vi "Autonomous Independent (Team 2175's conflicted copy 2013-08-08).vi"   [LabVIEW 2012]
doc: "This VI is called when autonomous begins, and will automatically be terminated when autonomous ends. You can carry out timed or sensor driven robot movement independently without needing to return to the caller."
uses:
  Robot Global Data.vi
  2013 Competition Code rev4 (Pre-Mariucci)/Auto Steer (Gyro).vi
types:
  T1 = typedef "WPI_GyroDevRef.ctl" = cluster{"DevStatus":errorcluster, "Analog Module":T2, "Analog Channel":T3, "Offset":dbl, "Gain (VoltsPerDegree/Second)":dbl}
  T2 = typedef "FPGA_TypedefAnalogModule.ctl" = enum16{"Analog Module 1", "Analog Module 2"}
  T3 = typedef "FPGA_AIChannel.ctl" = enum8{"AI 1", "AI 2", "AI 3", "AI 4", "AI 5", "AI 6", "AI 7", "AI 8", "Invalid"}
  T4 = typedef "WPI_EncoderDevRef.ctl" = cluster{"DevStatus":errorcluster, "EncoderIndex":T5, "CounterIndex":T6, "DistancePerCount":dbl, "Decoding Type":T7}
  T5 = typedef "FPGA_EncoderIdx.ctl" = enum8{"Enc 0", "Enc 1", "Enc 2", "Enc 3", "Invalid"}
  T6 = typedef "FPGA_CounterCtrSystemIndex.ctl" = enum8{"Ctr 0", "Ctr 1", "Ctr 2", "Ctr 3", "Ctr 4", "Ctr 5", "Ctr 6", "Ctr 7", "Invalid"}
  T7 = typedef "WPI_EncoderType.ctl" = enum16{"1x", "2x", "4x"}
  T8 = typedef "WPI_DigitalInputDevRef.ctl" = cluster{"DevStatus":errorcluster, "DIO Channel":T9, "Digital Module":T10}
  T9 = typedef "FPGA_DIOChannel.ctl" = enum8{"DIO 1", "DIO 2", "DIO 3", "DIO 4", "DIO 5", "DIO 6", "DIO 7", "DIO 8", "DIO 9", "DIO 10", "DIO 11", "DIO 12", "DIO 13", "DIO 14", "Invalid"}
  T10 = typedef "FPGA_TypedefDigitalModule.ctl" = enum16{"Digital Module 1", "Digital Module 2"}
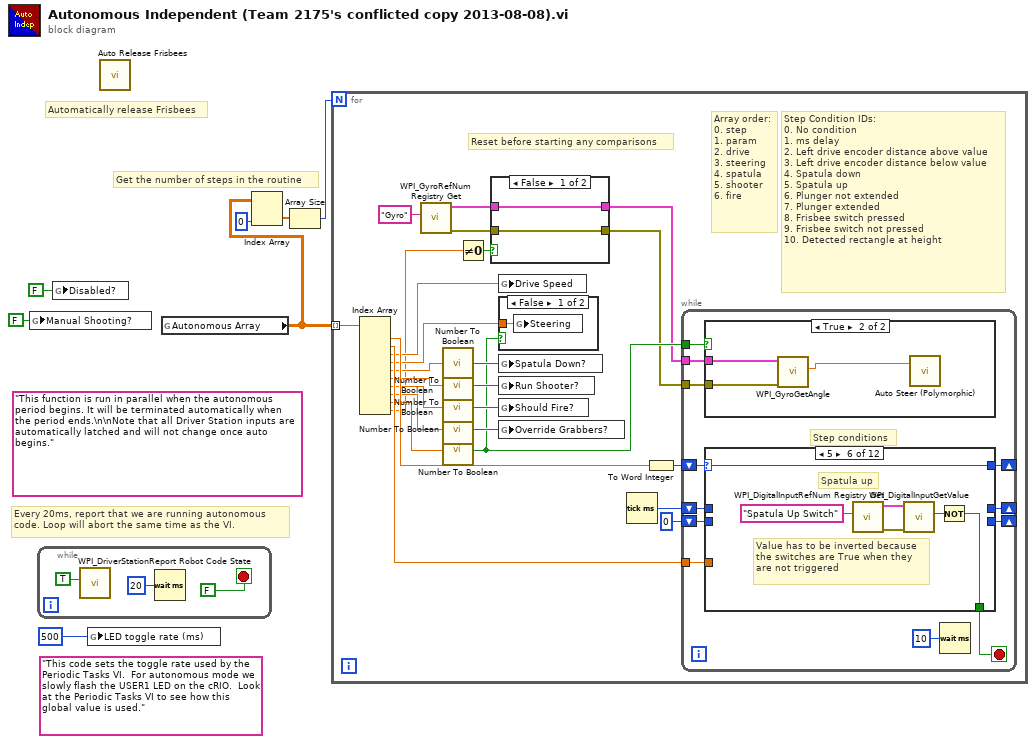
[diagram p0: block diagram]
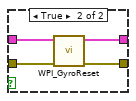
[diagram p2: hidden frame]
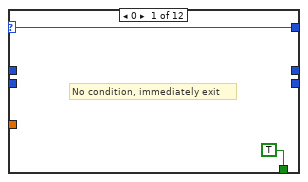
[diagram p5: hidden frame]
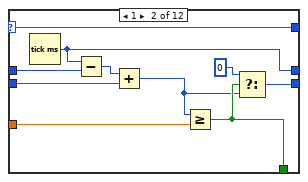
[diagram p6: hidden frame]
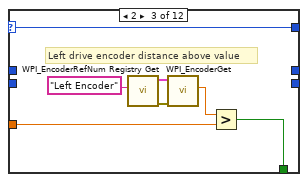
[diagram p7: hidden frame]
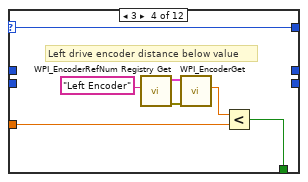
[diagram p8: hidden frame]
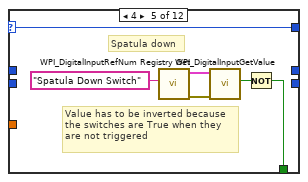
[diagram p9: hidden frame]
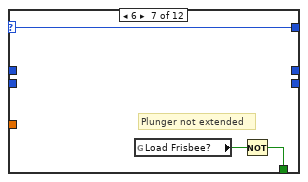
[diagram p10: hidden frame]
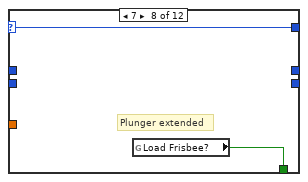
[diagram p11: hidden frame]
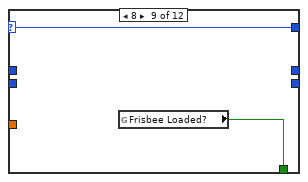
[diagram p12: hidden frame]
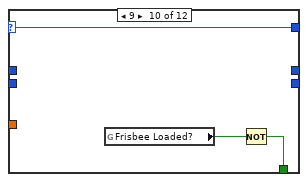
[diagram p13: hidden frame]
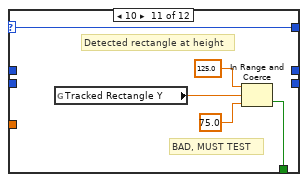
[diagram p14: hidden frame]
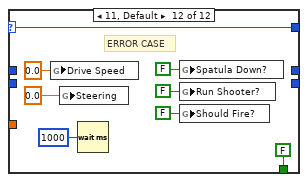
[diagram p15: hidden frame]
diagram:
  (unwired) "This code sets the toggle rate used by the Periodic Tasks VI.  For autonomous mode we slowly flash the USER1 LED on the cRIO.  Look at the Periodic Tasks VI to see how this global value is used."
  (unwired) "This function is run in parallel when the autonomous period begins. It will be terminated automatically when the period ends.\n\nNote that all Driver Station inputs are automatically latched and will not change once auto begins."
  # "Automatically release Frisbees"
  # "Get the number of steps in the routine"
  # "Every 20ms, report that we are running autonomous\ncode. Loop will abort the same time as the VI."
  n1 = global write "Robot Global Data.vi" "Manual Shooting?"(FALSE ("Disabled?")) -> ()
  n2 = while {
    stop <- FALSE stop-if-true
    n3 = call <vilib>:"WPI_DriverStationReport Robot Code State.vi"("Autonomous"=TRUE) -> ()  [unwired: 10 in, 1 out]
    n4 = Wait (ms)(milliseconds to wait=u32 20) -> ()  [unwired: 1 out]
  }
  n5 = global write "Robot Global Data.vi" "Disabled?"(FALSE ("Disabled?")) -> ()
  n6 = global write "Robot Global Data.vi" "LED toggle rate (ms)"(u32 500 ("LED ms toggle rate")) -> ()
  n7 = call "Auto Release Frisbees.vi"() -> ()  [unwired: 12 in]
  n8 = global read "Robot Global Data.vi" "Autonomous Array"() -> (w2:dbl[][])
  n9 = Index Array(array=w2, index (col)=0 ("disabled index (col)")) -> (element=w4:dbl[])  [unwired: 1 in]
  n10 = Array Size(array=w4) -> (size(s)=w5:i32)
  n11 = for {
    N: w5 -> [_]
    tunnel: w2 -> [w35] mode=indexing
    # "Reset before starting any comparisons"
    # "Array order:\n0. step\n1. param\n2. drive\n3. steering\n4. spatula\n5. shooter\n6. fire"
    # "Step Condition IDs:\n0. No condition\n1. ms delay\n2. Left drive encoder distance above value\n3. Left drive encoder distance below value\n4. Spatula down\n5. Spatula up\n6. Plunger not extended\n7. Plunger extended\n8. Frisbee switch pressed\n9. Frisbee switch not pressed\n10. Detected rectangle at height"
    n12 = Index Array(array=w35) -> (element #1=w33:dbl, element #2=w32:dbl, element #3=w22:dbl, element #4=w23:dbl, element #5=w31:dbl, element #6=w28:dbl, element #7=w26:dbl, element #8=w24:dbl, element #9=w21:dbl, element #10=w11:dbl)  [unwired: 10 in]
    n13 = call <vilib>:"WPI_GyroRefNum Registry Get.vi"("refnum name"="Gyro") -> ("error out"=w18:errorcluster, "GyroDevRef"=w17:T1)  [unwired: 9 in]
    n14 = call "Number To Boolean.vi"("Number"=w31) -> ("Boolean Value"=w30:bool)
    n15 = call "Number To Boolean.vi"("Number"=w28) -> ("Boolean Value"=w29:bool)
    n16 = call "Number To Boolean.vi"("Number"=w26) -> ("Boolean Value"=w27:bool)
    n17 = call "Number To Boolean.vi"("Number"=w24) -> ("Boolean Value"=w25:bool)
    n18 = call "Number To Boolean.vi"("Number"=w21) -> ("Boolean Value"=w20:bool)
    n19 = Not Equal To 0?(x=w11) -> (x != 0?=w12:bool)
    n20 = case shown="False" w12 {
      tunnel: w18 -> [w36 w41]
      tunnel: w17 -> [w37 w40]
      tunnel: [w37 w39] -> w16
      tunnel: [w36 w38] -> w15
      frame False {
      }
      frame True {
        n21 = call <vilib>:"WPI_GyroReset.vi"("error in (no error)"=w41, "GyroDevRef"=w40) -> ("error out"=w38:errorcluster, "GyroDevRef"=w39:T1)  [unwired: 8 in]
      }
    }
    n22 = global write "Robot Global Data.vi" "Drive Speed"(w22) -> ()
    n23 = case shown="False" w20 {
      tunnel: w23 -> [w42 _]
      frame False {
        n24 = global write "Robot Global Data.vi" "Steering"(w42) -> ()
      }
      frame True {
      }
    }
    n25 = global write "Robot Global Data.vi" "Spatula Down?"(w30) -> ()
    n26 = global write "Robot Global Data.vi" "Run Shooter?"(w29) -> ()
    n27 = global write "Robot Global Data.vi" "Should Fire?"(w27) -> ()
    n28 = global write "Robot Global Data.vi" "Override Grabbers?"(w25) -> ()
    n29 = Tick Count (ms)() -> (millisecond timer value=w14:u32)
    n30 = To Word Integer(number=w33) -> (16bit integer=w34:i16)
    n31 = while {
      shift-right: [w50] -> _
      shift-left: w34 -> [w54]
      tunnel: w32 -> [w52]
      tunnel: w20 -> [w49]
      tunnel: w16 -> [w48]
      tunnel: w15 -> [w47]
      shift-right: [w45] -> _
      shift-left: w14 -> [w46]
      shift-right: [w44] -> _
      shift-left: u32 0 -> [w43]
      stop <- w53 stop-if-true
      # "Step conditions"
      n32 = case shown="True" w49 {
        tunnel: w48 -> [_ w57]
        tunnel: w47 -> [_ w56]
        frame False {
        }
        frame True {
          n33 = call <vilib>:"WPI_GyroGetAngle.vi"("error in (no error)"=w56, "GyroDevRef"=w57) -> ("Angle"=w55:dbl)  [unwired: 6 in, 3 out]
          n34 = call-poly "Auto Steer (Polymorphic).vi"("Gyro Heading"=w55) -> ()  [unwired: 2 in]
        }
      }
      n35 = case shown="5" w54 {
        selector: w54 -> [w58 w69 w70 w77 w89 w95 w98 w100 w102 w104 w107 w111]
        tunnel: [TRUE w62 w71 w79 w84 w90 w96 w99 w101 w105 w110 FALSE] -> w53
        tunnel: w52 -> [_ w65 w72 w80 _ _ _ _ _ _ _ _]
        tunnel: [w58 w69 w70 w77 w89 w95 w98 w100 w102 w104 w107 w111] -> w50
        tunnel: w46 -> [_ w68 _ _ _ _ _ _ _ _ _ _]
        tunnel: [_ w67 _ _ _ _ _ _ _ _ _ _] -> w45
        tunnel: [_ w63 _ _ _ _ _ _ _ _ _ _] -> w44
        tunnel: w43 -> [_ w64 _ _ _ _ _ _ _ _ _ _]
        frame 0 {
          # "No condition, immediately exit"
        }
        frame 1 {
          n36 = Tick Count (ms)() -> (millisecond timer value=w67:u32)
          n37 = Subtract(x=w67, y=w68) -> (x-y=w66:u32)
          n38 = Add(x=w66, y=w64) -> (x+y=w60:u32)
          n39 = Greater Or Equal?(x=w60, y=w65) -> (x >= y?=w62:bool)
          n40 = Select(t=u32 0, s=w62, f=w60) -> (s? t:f=w63:u32)
        }
        frame 2 {
          # "Left drive encoder distance above value"
          n41 = call <vilib>:"WPI_EncoderRefNum Registry Get.vi"("refnum name"="Left Encoder") -> ("error out"=w74:errorcluster, "EncoderDevRef"=w75:T4)  [unwired: 9 in]
          n42 = call <vilib>:"WPI_EncoderGet.vi"("error in (no error)"=w74, "EncoderDevRef"=w75) -> ("Distance"=w73:dbl)  [unwired: 4 in, 5 out]
          n43 = Greater?(x=w73, y=w72) -> (0:w71:bool)
        }
        frame 3 {
          # "Left drive encoder distance below value"
          n44 = call <vilib>:"WPI_EncoderRefNum Registry Get.vi"("refnum name"="Left Encoder") -> ("error out"=w82:errorcluster, "EncoderDevRef"=w78:T4)  [unwired: 9 in]
          n45 = call <vilib>:"WPI_EncoderGet.vi"("error in (no error)"=w82, "EncoderDevRef"=w78) -> ("Distance"=w81:dbl)  [unwired: 4 in, 5 out]
          n46 = Less?(x=w81, y=w80) -> (x < y?=w79:bool)
        }
        frame 4 {
          # "Value has to be inverted because\nthe switches are True when they\nare not triggered"
          # "Spatula down"
          n47 = call <vilib>:"WPI_DigitalInputRefNum Registry Get.vi"("refnum name"="Spatula Down Switch") -> ("error out"=w87:errorcluster, "DigitalInputDevRef"=w86:T8)  [unwired: 9 in]
          n48 = call <vilib>:"WPI_DigitalInputGetValue.vi"("error in (no error)"=w87, "DigitalInputDevRef"=w86) -> ("Value"=w85:bool)  [unwired: 7 in, 2 out]
          n49 = Not(x=w85) -> (.not. x?=w84:bool)
        }
        frame 5 {
          # "Value has to be inverted because\nthe switches are True when they\nare not triggered"
          # "Spatula up"
          n50 = call <vilib>:"WPI_DigitalInputRefNum Registry Get.vi"("refnum name"="Spatula Up Switch") -> ("error out"=w93:errorcluster, "DigitalInputDevRef"=w92:T8)  [unwired: 9 in]
          n51 = call <vilib>:"WPI_DigitalInputGetValue.vi"("error in (no error)"=w93, "DigitalInputDevRef"=w92) -> ("Value"=w91:bool)  [unwired: 7 in, 2 out]
          n52 = Not(x=w91) -> (.not. x?=w90:bool)
        }
        frame 6 {
          # "Plunger not extended"
          n53 = global read "Robot Global Data.vi" "Load Frisbee?"() -> (w97:bool)
          n54 = Not(x=w97) -> (.not. x?=w96:bool)
        }
        frame 7 {
          # "Plunger extended"
          n55 = global read "Robot Global Data.vi" "Load Frisbee?"() -> (w99:bool)
        }
        frame 8 {
          n56 = global read "Robot Global Data.vi" "Frisbee Loaded?"() -> (w101:bool)
        }
        frame 9 {
          n57 = global read "Robot Global Data.vi" "Frisbee Loaded?"() -> (w103:bool)
          n58 = Not(x=w103) -> (.not. x?=w105:bool)
        }
        frame 10 {
          # "BAD, MUST TEST"
          # "Detected rectangle at height"
          n59 = global read "Robot Global Data.vi" "Tracked Rectangle Y"() -> (w106:dbl)
          n60 = In Range and Coerce(upper limit=125.0, x=w106, lower limit=75.0) -> (In Range?=w110:bool)  [unwired: 1 out]
        }
        frame 11, Default {
          # "ERROR CASE"
          n61 = global write "Robot Global Data.vi" "Drive Speed"(0.0 ("Drive Speed")) -> ()
          n62 = global write "Robot Global Data.vi" "Steering"(0.0 ("Drive Speed")) -> ()
          n63 = Wait (ms)(milliseconds to wait=u32 1000) -> ()  [unwired: 1 out]
          n64 = global write "Robot Global Data.vi" "Spatula Down?"(FALSE ("Spatula Down?")) -> ()
          n65 = global write "Robot Global Data.vi" "Run Shooter?"(FALSE ("Run Shooter?")) -> ()
          n66 = global write "Robot Global Data.vi" "Should Fire?"(FALSE ("Should Fire?")) -> ()
        }
      }
      n67 = Wait (ms)(milliseconds to wait=u32 10) -> ()  [unwired: 1 out]
    }
  }
